vi "Run_JumboBooks.vi"   [LabVIEW 2012]
panel:
  # "Launching JumboBooks"
types:
  T1 = enum32{"Invalid", "Standard", "Closed", "Hidden", "Minimized", "Maximized"}
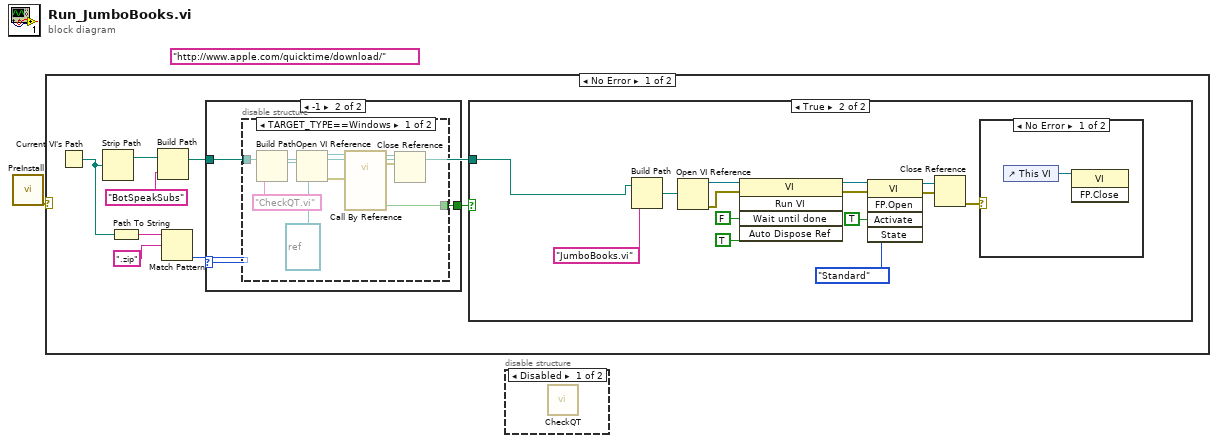
[diagram p0: block diagram]
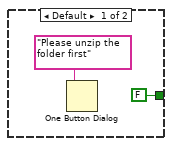
[diagram p5: hidden frame]
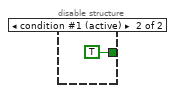
[diagram p6: hidden frame]
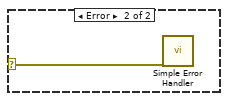
[diagram p7: hidden frame]
diagram:
  (unwired) "http://www.apple.com/quicktime/download/" ("regular expression")
  n1 = call "PreInstall.vi"() -> ("error out"=w1:errorcluster)  [unwired: 3 in]
  n2 = case shown="No Error" w1 {
    selector: w1 -> [_ w39]
    frame No Error {
      n3 = Current VI's Path() -> (path=w3:path)
      n4 = Strip Path(path=w3) -> (stripped path=w4:path)  [unwired: 1 out]
      n5 = Path To String(path=w3) -> (string=w9:string)
      n6 = Build Path(base path=w4, name or relative path="BotSpeakSubs") -> (appended path=w2:path)
      n7 = Match Pattern(string=w9, regular expression=".zip") -> (offset past match=w7:i32)  [unwired: 1 in, 3 out]
      n8 = case shown="-1" w7 {
        tunnel: [FALSE w28] -> w6
        tunnel: w2 -> [_ w27]
        frame Default {
          n9 = One Button Dialog(message="Please unzip the folder first") -> ()  [unwired: 1 in, 1 out]
        }
        frame -1 {
          n10 = disable-structure shown="TARGET_TYPE==Windows" {
            disable-tunnel: [w32 TRUE] -> w28
            disable-tunnel: w27 -> [w37 _]
            frame condition #0 {
              n11 = Build Path(base path=w37, name or relative path="CheckQT.vi" ("regular expression")) -> (appended path=w29:path)
              n12 = Open VI Reference(type specifier VI Refnum (for type only)=refnum<vi> refnum, vi path=w29) -> (vi reference=w35:refnum<vi>, error out=w34:errorcluster)  [unwired: 4 in]
              n13 = call-by-ref "?"(reference=w35, error in=w34) -> (reference out=w31:refnum<vi>, error out=w30:errorcluster, "success?"=w32:bool)  [unwired: 3 in]
              n14 = Close Reference(reference=w31, error in (no error)=w30) -> ()  [unwired: 1 out]
            }
            frame condition #1 (active) {
            }
          }
        }
      }
      n15 = case shown="True" w6 {
        tunnel: w2 -> [_ w10]
        frame False {
        }
        frame True {
          n16 = Build Path(base path=w10, name or relative path="JumboBooks.vi") -> (appended path=w22:path)
          n17 = Open VI Reference(vi path=w22) -> (vi reference=w21:refnum<vi>, error out=w20:errorcluster)  [unwired: 5 in]
          n18 = invoke class="VI" method="Run VI"(reference=w21, error in=w20, "Wait until done"=FALSE ("Wait Until Done"), "Auto Dispose Ref"=TRUE ("Auto Dispose Reference")) -> (reference out=w16:refnum<vi>, error out=w15:errorcluster)  [unwired: 1 in, 3 out]
          n19 = invoke class="VI" method="FP.Open"(reference=w16, error in=w15, "Activate"=TRUE ("Activate?"), "State"=T1."Standard") -> (reference out=w13:refnum<vi>, error out=w14:errorcluster)  [unwired: 1 in, 3 out]
          n20 = Close Reference(reference=w13, error in (no error)=w14) -> (error out=w17:errorcluster)
          n21 = case shown="No Error" w17 {
            frame No Error {
              n22 = control-ref of="This VI"() -> (w24:refnum<vi>)
              n23 = invoke class="VI" method="FP.Close"(reference=w24) -> ()  [unwired: 2 in, 3 out]
            }
            frame Error {
            }
          }
        }
      }
    }
    frame Error {
      n24 = call <vilib>:"Simple Error Handler.vi"("error in (no error)"=w39) -> ()  [unwired: 4 in, 5 out]
    }
  }
  n25 = disable-structure shown="Disabled" {
    frame Disabled {
      n26 = call "CheckQT.vi"() -> ()  [unwired: 3 in, 1 out]
    }
    frame Enabled {
    }
  }
